vi "field-raster-globals.vi"() -> ()   [LabVIEW 2014]
uses:
  small z increment.ctl
panel:
  in  "check":dbl
  in  "YFieldDown":u32
  in  "XFieldDiff":dbl
  in  "YFieldUp":u32
  in  "current Y":dbl
  in  "current X":dbl
  in  "Previous small Z increment":T1
  in  "Zmax":dbl
  in  "Xmax":dbl
  in  "Ymax":dbl
  out "Plot2":cluster{dbl[], dbl[]}={[0.0, 200.0], [200.0, 200.0]}
  out "Plot1":cluster{dbl[], dbl[]}={[0.0, 200.0], [0.0, 0.0]}
  in  "Y mark down":dbl
  in  "Y mark up":dbl
  in  "X mark down":dbl
  in  "X mark up":dbl
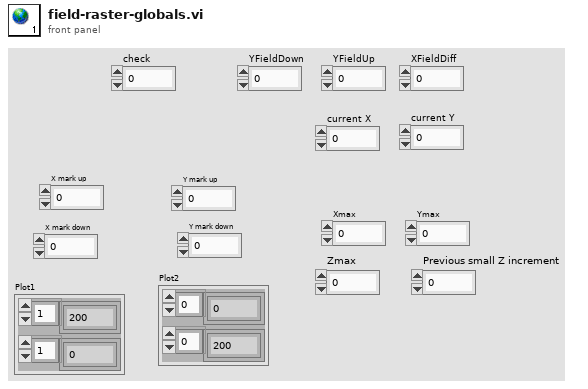
[diagram p1: front panel]
types:
  T1 = typedef "small z increment.ctl" = dbl
diagram:
